vi "read database.vi"(10 "database cluster write data in 3":T1={"ID"=0, "Datetime"="17-03-2020 14:45:50", "PARTBARCODE"="", "TORQUE"="", "RESULT1"="", "CHILD1"="", "CHILD2"="A1234567B567003", "CHILD3"="", "CHILD4"="", "RESULT2"="OK", "FINALBARCODE"="", "RESULT3"="", "REMARK"="", "OTHER"=""}, 11 "Data Read":variant[][](array[variant])) -> (0 "database cluster Read":T1, 1 "Barcode not Found":bool, 3 "database cluster write data":T1={"ID"=0, "Datetime"="17-03-2020 14:45:50", "PARTBARCODE"="", "TORQUE"="", "RESULT1"="", "CHILD1"="", "CHILD2"="A1234567B567003", "CHILD3"="", "CHILD4"="", "RESULT2"="OK", "FINALBARCODE"="", "RESULT3"="", "REMARK"="", "OTHER"=""}, 4 "Rework Part @ station 1":bool, 5 "Dispalya":string[](array[string]), 7 "Search result":string[][](table))   [LabVIEW 2024]
uses:
  database cluster.ctl
  <vilib>/addons/database/_DB Variant To Data/Database Variant To Data.xnode
panel:
  out "ID":i32
  out "element":i32
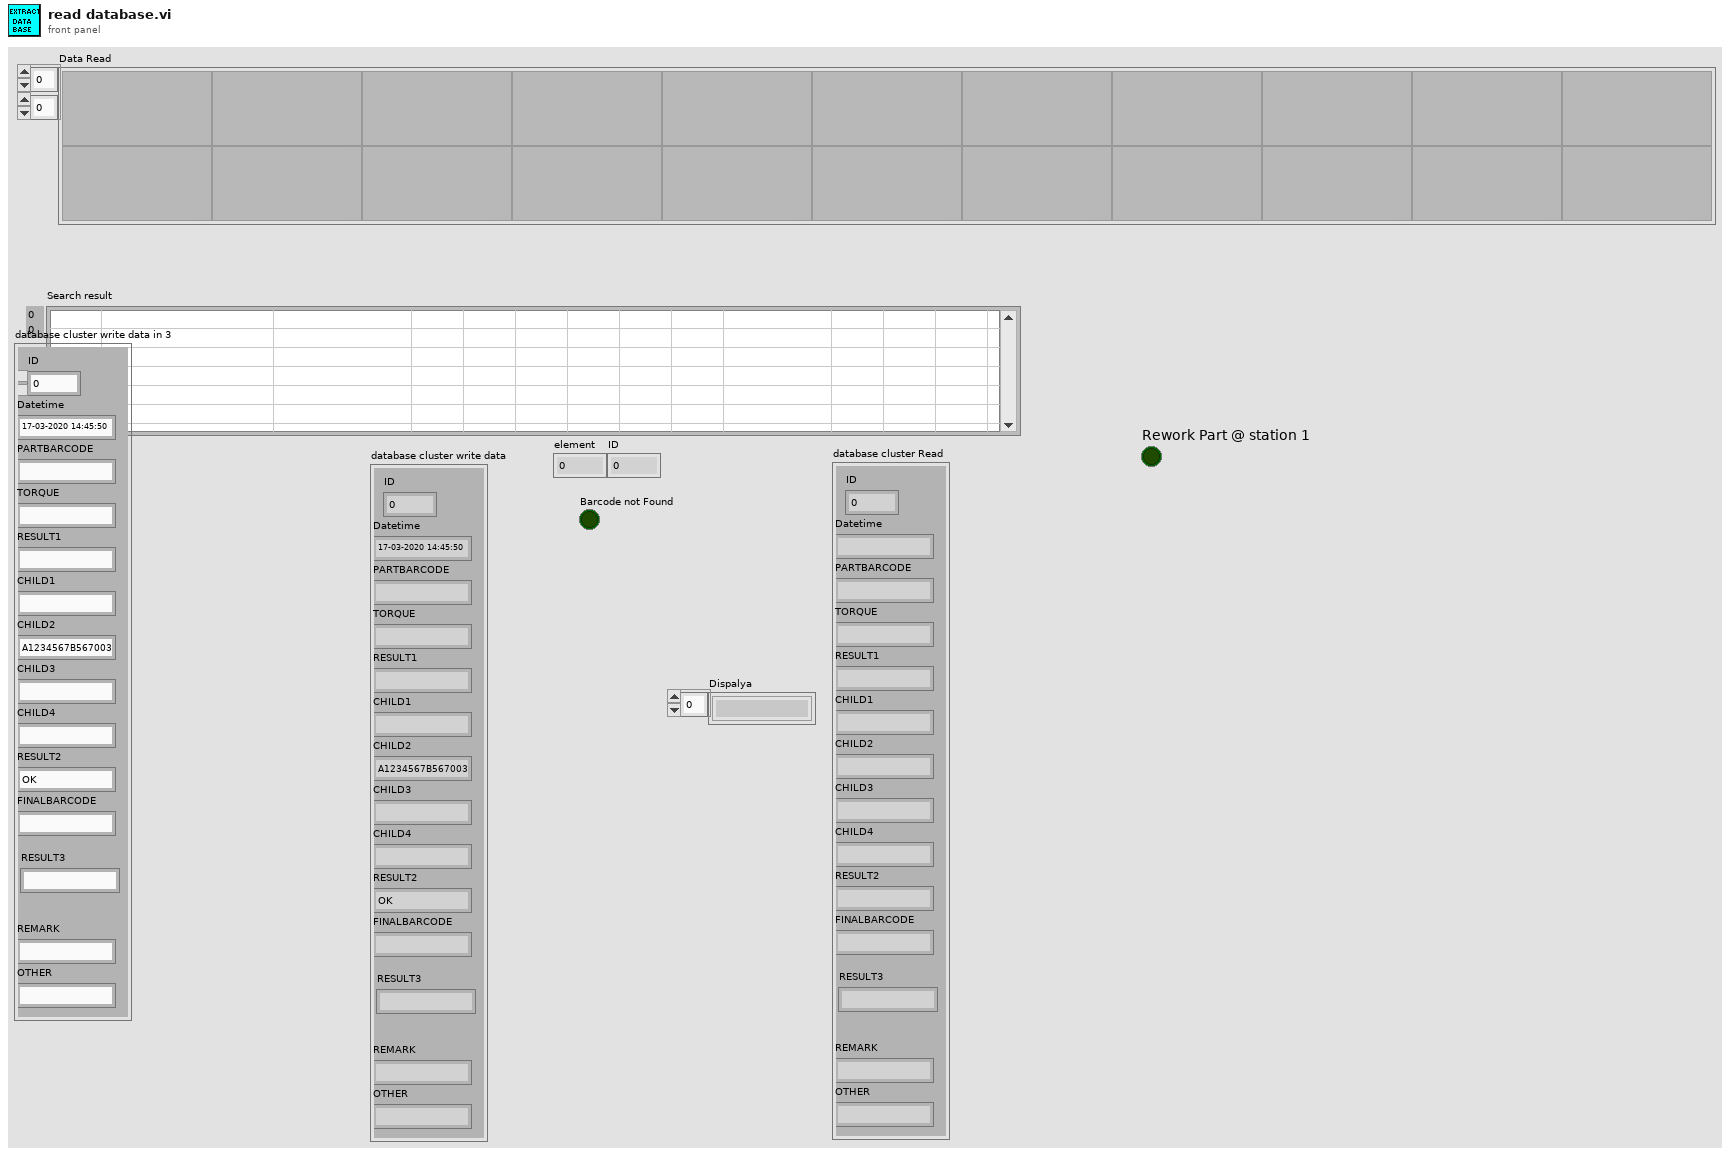
[diagram p1: front panel]
types:
  T1 = typedef "database cluster.ctl" = cluster{"ID":i64, "Datetime":string, "PARTBARCODE":string, "TORQUE":string, "RESULT1":string, "CHILD1":string, "CHILD2":string, "CHILD3":string, "CHILD4":string, "RESULT2":string, "FINALBARCODE":string, "RESULT3":string, "REMARK":string, "OTHER":string}
  T2 = cluster{"data[0]":string, "data[1]":string, "data[2]":string, "data[3]":string, "data[4]":string, "data[5]":string, "data[6]":string, "data[7]":string, "data[8]":string, "data[9]":string, "data[10]":string, "data[11]":string, "data[12]":string, "data[13]":string, "data[14]":string}
  T3 = cluster{i32, "Datetime":string, "PARTBARCODE":string, "TORQUE":string, "RESULT1":string, "CHILD1":string, "CHILD2":string, "CHILD3":string, "CHILD4":string, "RESULT2":string, "FINALBARCODE":string, "RESULT3":string, "REMARK":string, "OTHER":string}
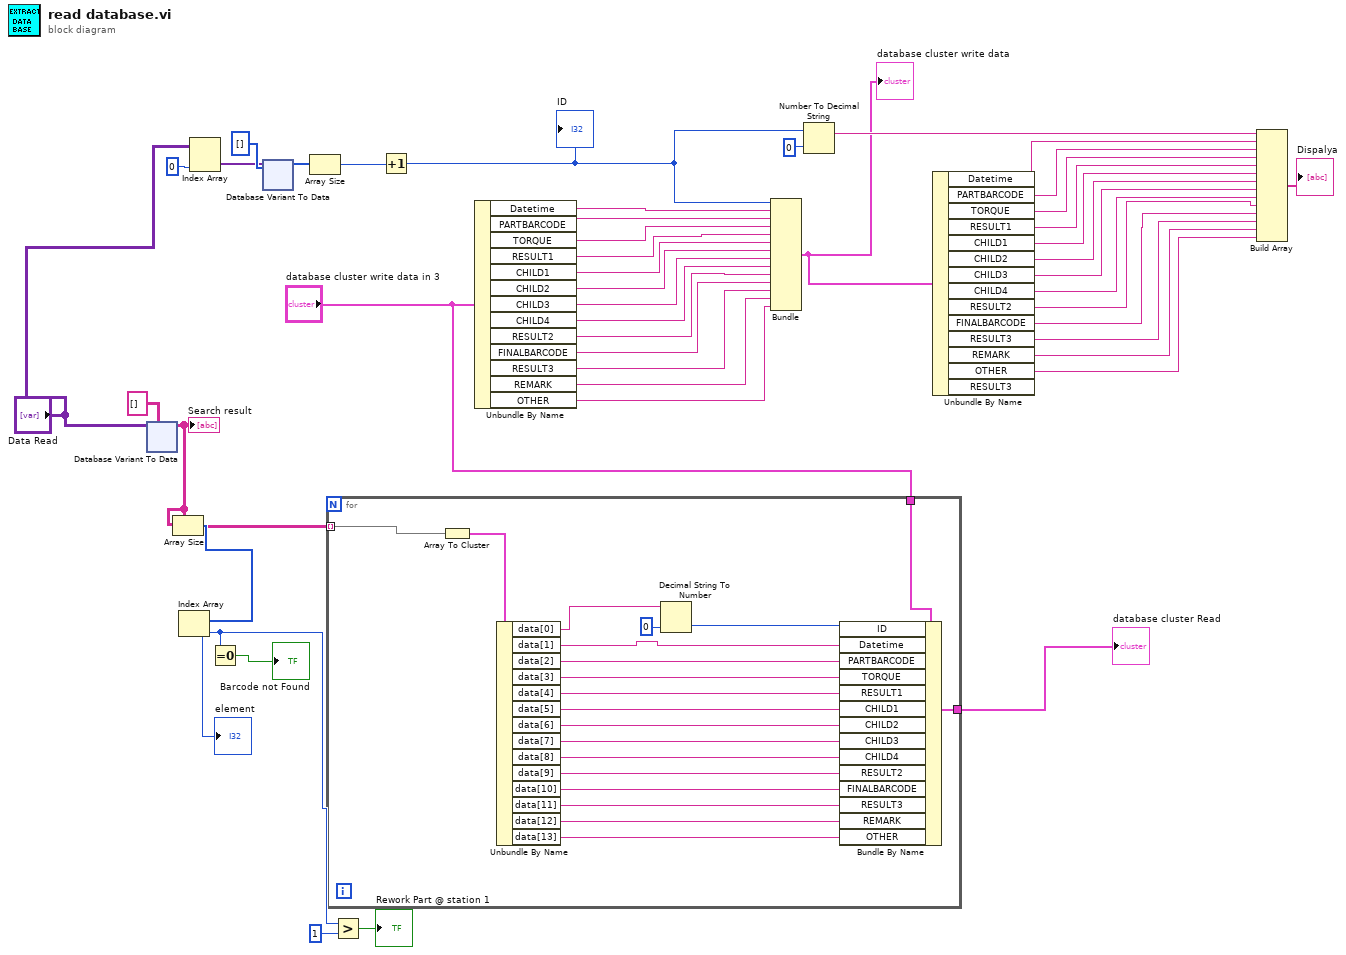
[diagram p0: block diagram]
diagram:
  n1 = xnode "Database Variant To Data"("database variant"="Data Read", "type"=string[][] [] ("Array")) -> ("data"=w44:string[][])  [unwired: 1 in, 1 out]
  "Search result" <- w44
  n2 = Array Size(array=w44) -> (size(s)=w45:i32[])
  n3 = Index Array(array=w45) -> (element=w8:i32)  [unwired: 1 in]
  "element" <- w8
  n4 = Index Array(array="Data Read", index (col)=0 ("disabled index (col)")) -> (element=w40:variant[])  [unwired: 1 in]
  n5 = Equal To 0?(x=w8) -> (x = 0?=→"Barcode not Found":bool)
  n6 = xnode "Database Variant To Data"("database variant"=w40, "type"=i64[] []) -> ("data"=w41:i64[])  [unwired: 1 in, 1 out]
  n7 = Array Size(array=w41) -> (size(s)=w43:i32)
  n8 = for {
    tunnel: w44 -> [w62] mode=indexing
    tunnel: "database cluster write data in 3" -> [w61]
    tunnel: [w60] -> w4
    n9 = Array To Cluster(array=w62) -> (cluster=w66:T2)
    n10 = Unbundle By Name(w66) -> ("data[0]"=w64:string, "data[1]"=w63:string, "data[2]"=w59:string, "data[3]"=w58:string, "data[4]"=w57:string, "data[5]"=w56:string, "data[6]"=w55:string, "data[7]"=w54:string, "data[8]"=w53:string, "data[9]"=w52:string, "data[10]"=w51:string, "data[11]"=w50:string, "data[12]"=w49:string, "data[13]"=w48:string)
    n11 = Decimal String To Number(string=w64, default (0L)=i64 0) -> (number=w47:i64)  [unwired: 1 in, 1 out]
    n12 = Bundle By Name(cluster=w61, "ID"=w47, "Datetime"=w63, "PARTBARCODE"=w59, "TORQUE"=w58, "RESULT1"=w57, "CHILD1"=w56, "CHILD2"=w55, "CHILD3"=w54, "CHILD4"=w53, "RESULT2"=w52, "FINALBARCODE"=w51, "RESULT3"=w50, "REMARK"=w49, "OTHER"=w48) -> (w60:T1)
  }
  "database cluster Read" <- w4
  n13 = Greater?(x=w8, y=1) -> (0:→"Rework Part @ station 1":bool)
  n14 = Increment(x=w43) -> (x+1=w12:i32)
  "ID" <- w12
  n15 = Unbundle By Name("database cluster write data in 3") -> ("Datetime"=w11:string, "PARTBARCODE"=w18:string, "TORQUE"=w38:string, "RESULT1"=w37:string, "CHILD1"=w36:string, "CHILD2"=w35:string, "CHILD3"=w34:string, "CHILD4"=w24:string, "RESULT2"=w23:string, "FINALBARCODE"=w22:string, "RESULT3"=w16:string, "REMARK"=w14:string, "OTHER"=w1:string)
  n16 = Bundle(w12, "Datetime"=w11, "PARTBARCODE"=w18, "TORQUE"=w38, "RESULT1"=w37, "CHILD1"=w36, "CHILD2"=w35, "CHILD3"=w34, "CHILD4"=w24, "RESULT2"=w23, "FINALBARCODE"=w22, "RESULT3"=w16, "REMARK"=w14, "OTHER"=w1) -> (w3:T3)  [unwired: 1 in]
  "database cluster write data" <- w3
  n17 = Number To Decimal String(number=w12, width (-)=i64 0) -> (decimal integer string=w17:string)
  n18 = Unbundle By Name(w3) -> ("Datetime"=w9:string, "PARTBARCODE"=w10:string, "TORQUE"=w31:string, "RESULT1"=w30:string, "CHILD1"=w29:string, "CHILD2"=w28:string, "CHILD3"=w27:string, "CHILD4"=w21:string, "RESULT2"=w20:string, "FINALBARCODE"=w19:string, "RESULT3"=w15:string, "REMARK"=w13:string, "OTHER"=w2:string)  [unwired: 1 out]
  n19 = Build Array(w17, w9, w10, w31, w30, w29, w28, w27, w21, w20, w19, w15, w13, w2) -> (→"Dispalya":string[])
